vi "Rough TDMS Viewer.vi"() -> ()   [LabVIEW 2019, in "Report Viewer.lvlib" / "Report Viewer.lvclass"]
doc: "Defer all the request for panel update the panel list. This will improve the loading time."
uses:
  Report Viewer.lvclass
  Custom Controls/Browse Tools.ctl
  <vilib>/Utility/tdmsutil.llb/fileViewerConfigData.ctl
panel:
  out "TDMS File":string="Please using \"OPEN TDMS\" button to select tdms file."
  in  "Display Format":T1(ring)
  in  "Settings":bool
  in  "Properties / Values / Graph":T2(tab)=enum."Analog values (graph)"
  in  "Properties":i32(listbox)
  in  "Raw data values":i32(listbox)=-1
  out "Delta X (Time mS)":dbl
  out "Waveform Graph":waveform(dbl)[](graph)=[{"t0"=timestamp(0 s since 1904-01-01), "dt"=1.0, "Y"=[]}]
  out "Delta Y (Amplitude)":dbl
  in  "File contents":string[](tree)=["\"\u0000\u0000\u0000\u0002\u0000\u0000\u0000+Halt Mode Running_11:25:18.755 AM 11/6/2019\u0000\u0000\u0000\nPJB1_S CH0\""]
  in  "Open TDMS":bool
  in  "Save Graph":bool
  in  "Save Data":bool
  in  "Finished":bool
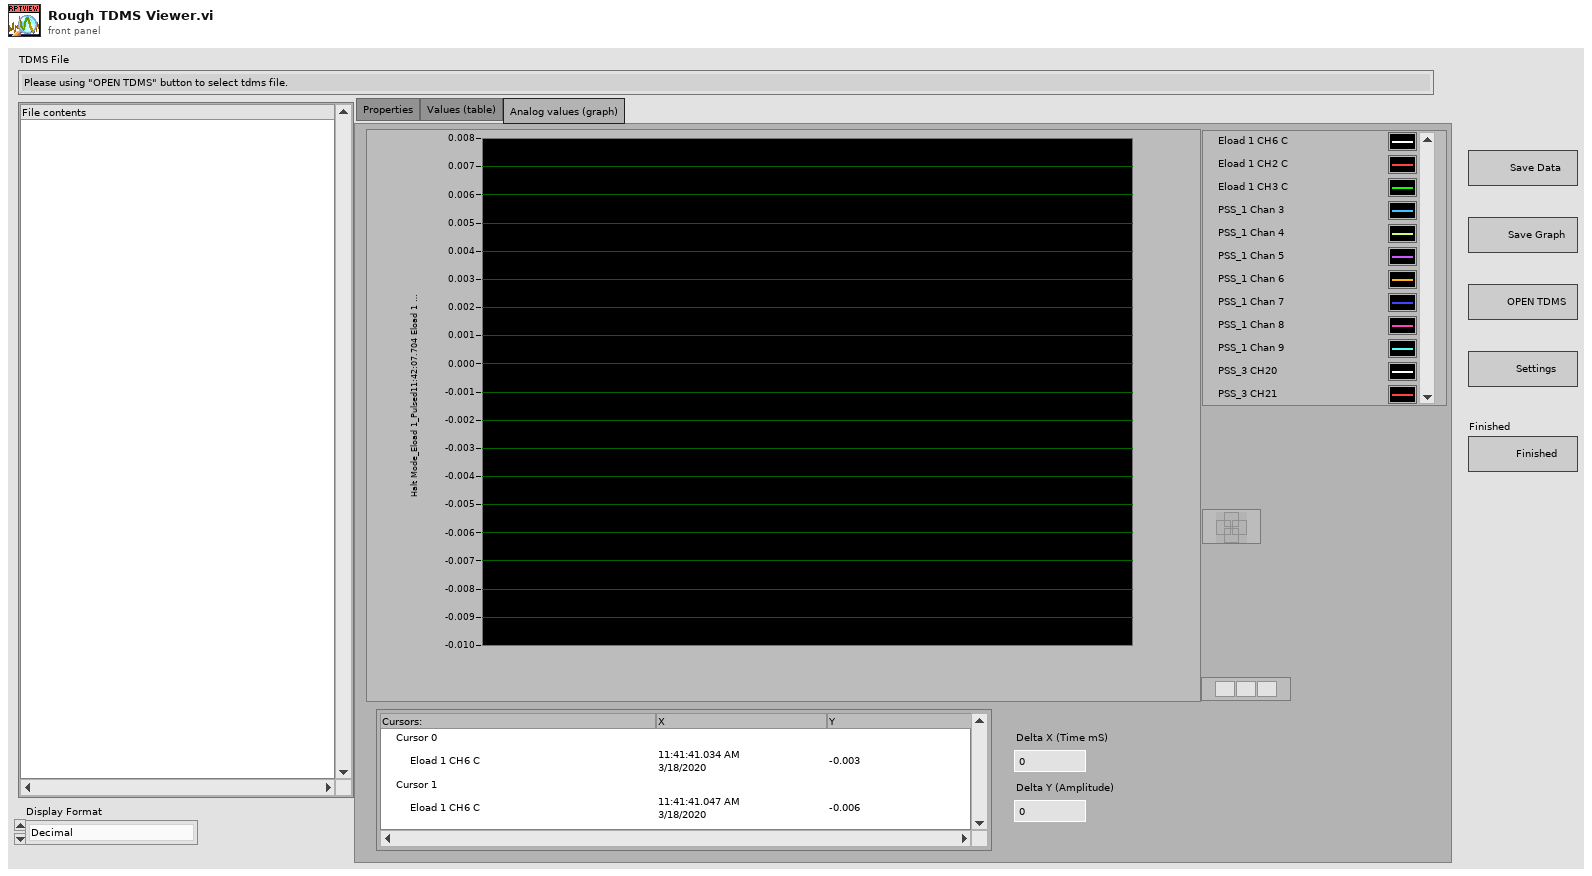
[diagram p1: front panel]
types:
  T1 = enum16{"Decimal", "Scientific", "Engineering", "Binary", "Octal", "Hexadecimal"}
  T2 = enum32{"Properties", "Values (table)", "Analog values (graph)"}
  T3 = enum32{"Invalid", "Standard", "Closed", "Hidden", "Minimized", "Maximized"}
  T4 = typedef "fileViewerConfigData.ctl" = cluster{"Show all (table)":bool, "Show all (graph)":bool, "limit (table)":u64, "limit (graph)":u64, "no show":bool, "start (table)":u64, "start (graph)":u64}
  T5 = typedef "Report Viewer.lvlib/Report Viewer.lvclass/Browse Tools.ctl" = cluster{"Group":string, "Channel":string, "TDMS View Cfg":T4}
  T6 = typedef "imagedata.ctl" = cluster{"image type":i32, "image depth":i32, "image":u8[], "mask":u8[], "colors":u32[], "Rectangle":cluster{"left":i16, "top":i16, "right":i16, "bottom":i16}}
  T7 = typedef "LVCursorListTypeDef.ctl" = cluster{"Name":string, "Color":u32, "Style":u8, "Point Style":u8, "Name Visible":bool, "Allow Drag":bool, "Cursor Mode":u32, "Plot":i32, "Index":i32, "Position":cluster{"X":dbl, "Y":dbl}, "X Scale":u32, "Y Scale":u32, "Watch Plots":i32[], "Watch All Plots":bool, "Plot Area":i32, "Label Offset":cluster{"X":dbl, "Y":dbl}}[]
  T8 = cluster{"Name":string, "Color":u32, "Style":u8, "Point Style":u8, "Name Visible":bool, "Allow Drag":bool, "Cursor Mode":u32, "Plot":i32, "Index":i32, "Position":cluster{"X":dbl, "Y":dbl}, "X Scale":u32, "Y Scale":u32, "Watch Plots":i32[], "Watch All Plots":bool, "Plot Area":i32, "Label Offset":cluster{"X":dbl, "Y":dbl}}
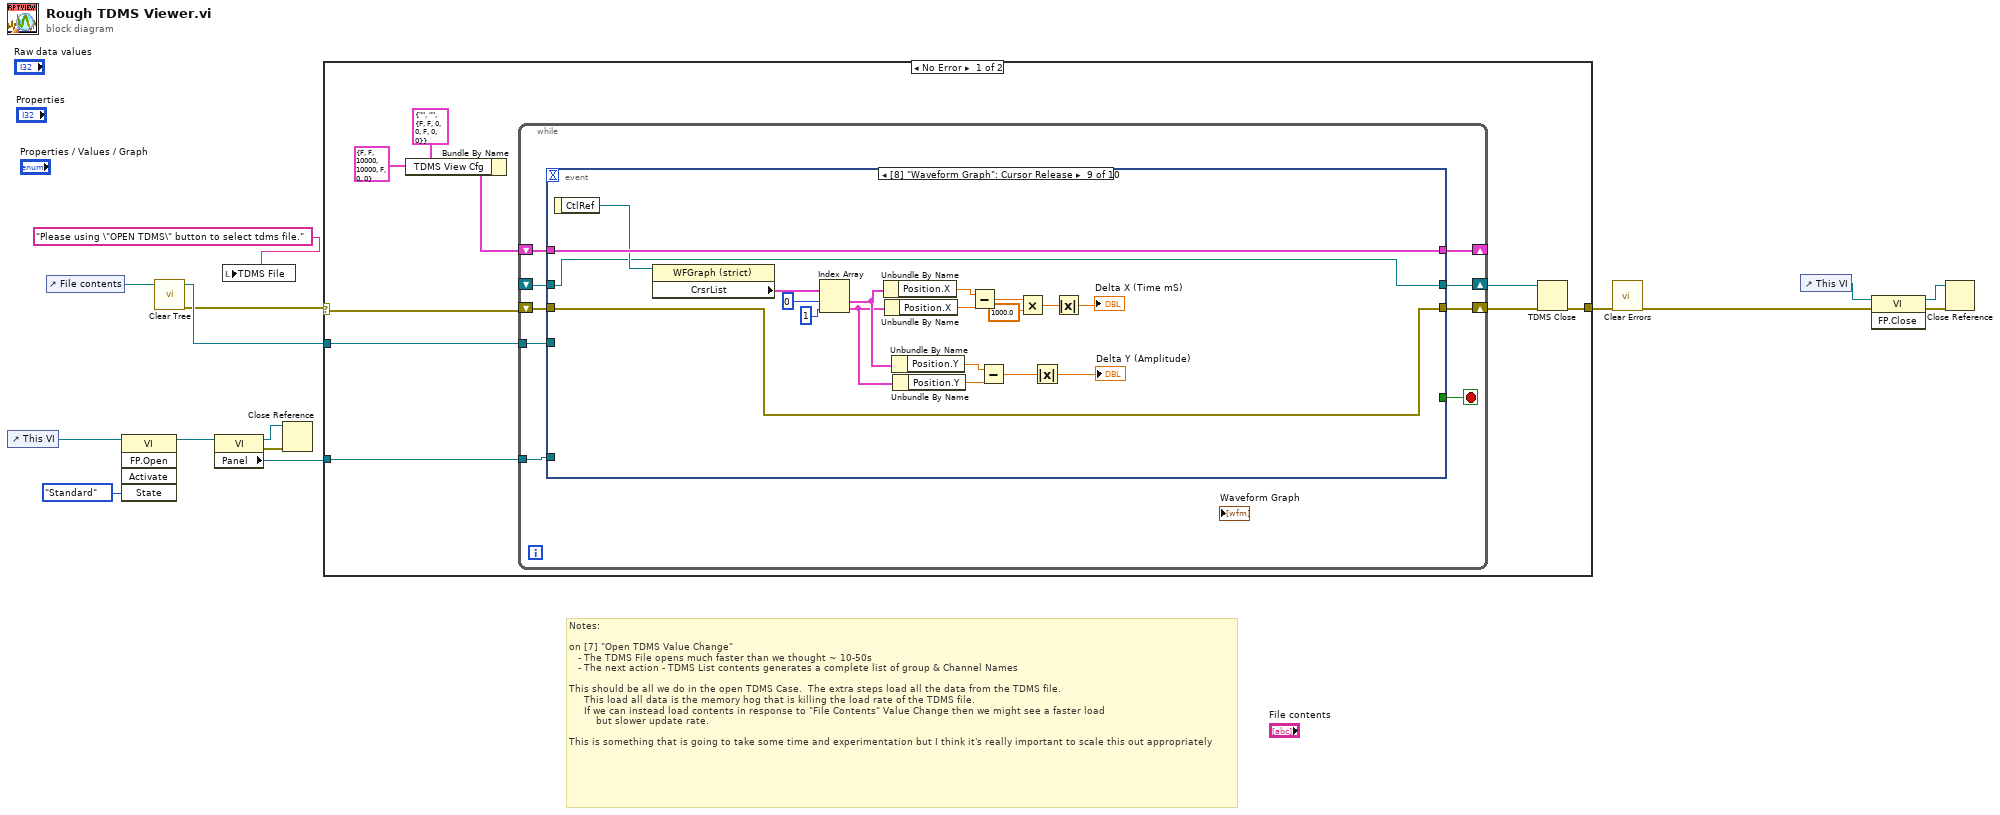
[diagram p0: block diagram]
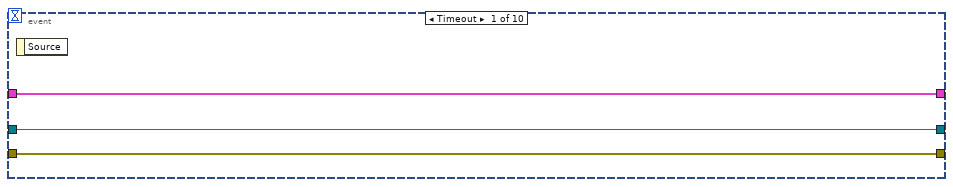
[diagram p2: hidden frame]
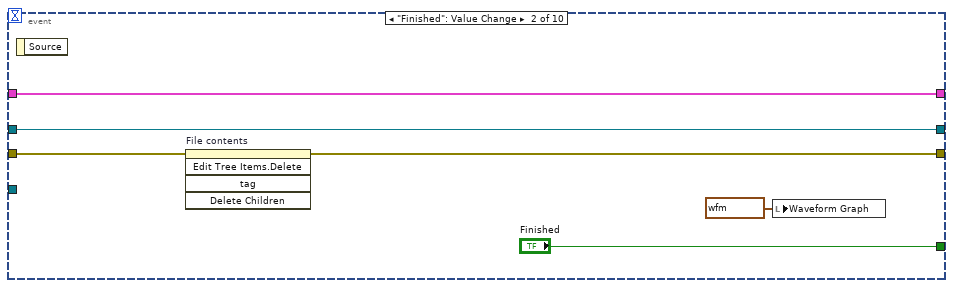
[diagram p3: hidden frame]
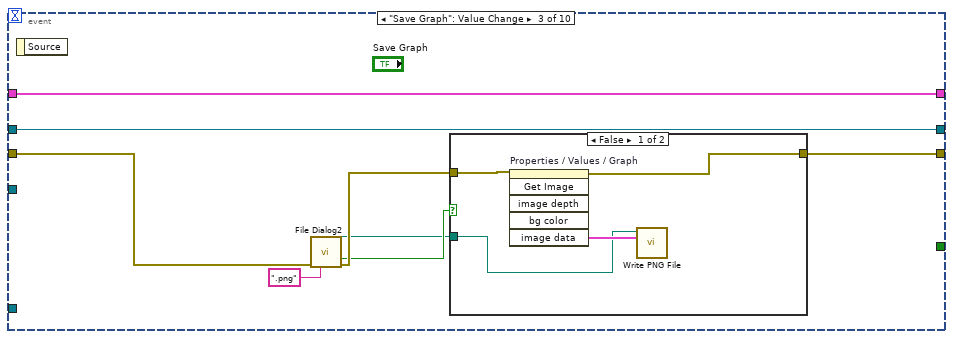
[diagram p4: hidden frame]
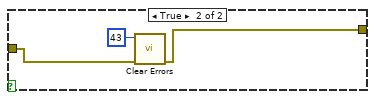
[diagram p5: hidden frame]
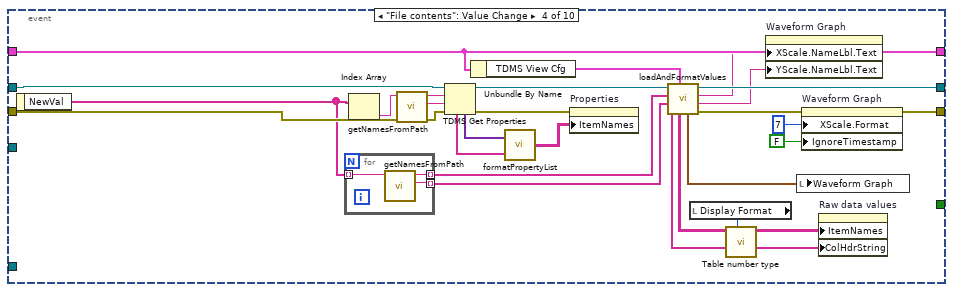
[diagram p6: hidden frame]
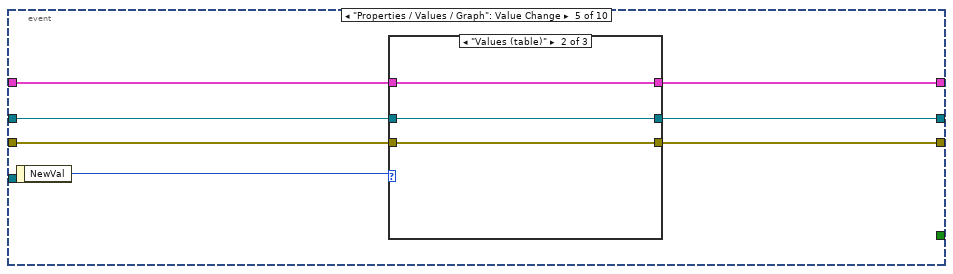
[diagram p7: hidden frame]
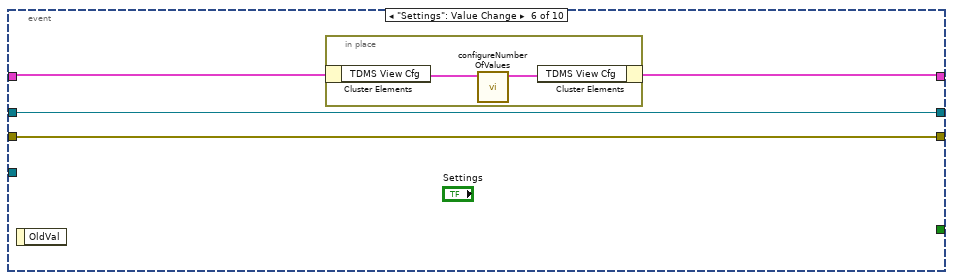
[diagram p10: hidden frame]
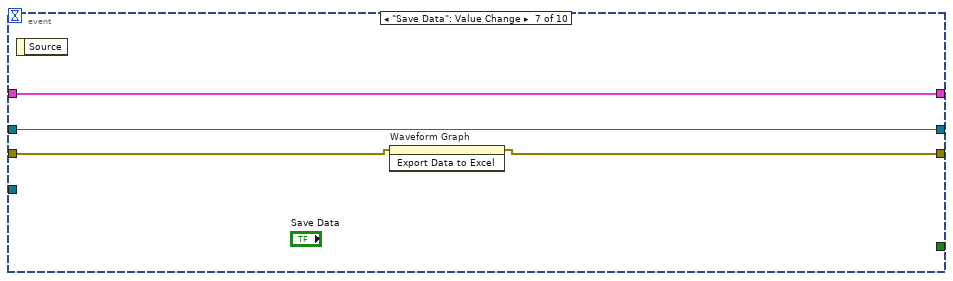
[diagram p11: hidden frame]
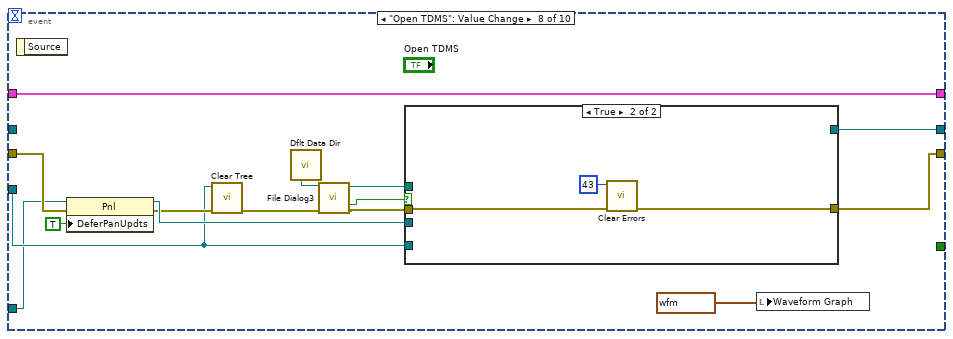
[diagram p12: hidden frame]
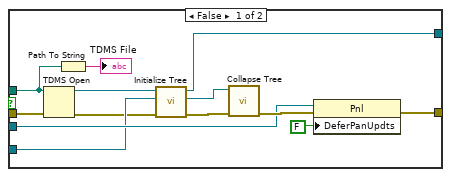
[diagram p13: hidden frame]
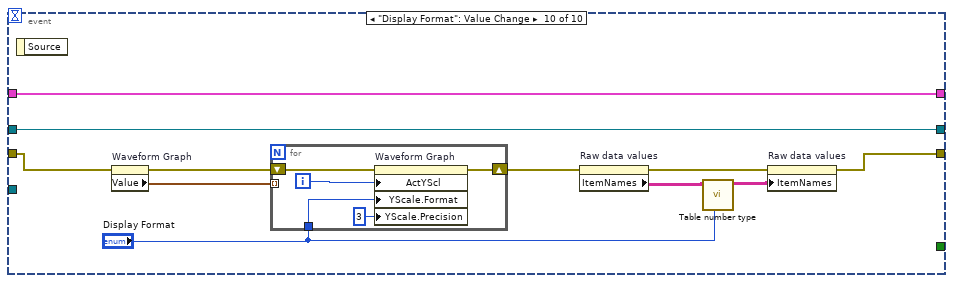
[diagram p14: hidden frame]
diagram:
  # "Notes:\n\non [7] \"Open TDMS Value Change\"\n   - The TDMS File opens much faster than we thought ~ 10-50s\n   - The next action - TDMS List contents generates a complete list of group & Channel Names\n\nThis should be all we do in the open TDMS Case.  The extra steps load all the data from the TDMS file.\n     This load all data is the memory hog that is killing the load rate of the TDMS file.  \n     If we can instead load contents in response to \"File Contents\" Value Change then we might see a faster load\n         but slower update rate.  \n\nThis is something that is going to take some time and experimentation but I think it's really important to scale this out appropriately"
  n1 = control-ref of="This VI"() -> (w13:refnum<vi>)
  n2 = control-ref of="File contents"() -> (w10:refnum<vi>)
  n3 = invoke class="VI" method="FP.Open"(reference=w13, "State"=T3."Standard") -> (reference out=w5:refnum<vi>)  [unwired: 3 in, 4 out]
  n4 = call "Clear Tree.vi"("reference"=w10) -> ("error out"=w8:errorcluster, "reference out"=w9:refnum<vi>)  [unwired: 9 in]
  n5 = property class="VI"(reference=w5) -> (reference out=w11:refnum<vi>, error out=w12:errorcluster, "Panel"=w6:refnum<vi>)  [unwired: 1 in]
  n6 = local write "TDMS File"("Please using \"OPEN TDMS\" button to select tdms file.") -> ()
  n7 = Close Reference(reference=w11, error in (no error)=w12) -> ()  [unwired: 1 out]
  n8 = case shown="No Error" w8 {
    selector: w8 -> [w17 w180]
    tunnel: [w24 w180] -> w15
    tunnel: w9 -> [w19 _]
    tunnel: w6 -> [w16 _]
    frame No Error {
      n9 = Bundle By Name(cluster=T5 {"Group"="", "Channel"="", "TDMS View Cfg"={"Show all (table)"=FALSE, "Show all (graph)"=FALSE, "limit (table)"=0, "limit (graph)"=0, "no show"=FALSE, "start (table)"=0, "start (graph)"=0}} ("Cluster"), "TDMS View Cfg"=T4 {"Show all (table)"=FALSE, "Show all (graph)"=FALSE, "limit (table)"=10000, "limit (graph)"=10000, "no show"=FALSE, "start (table)"=0, "start (graph)"=0} ("TDMS File Viewer Configuration")) -> (w21:T5)
      n10 = while {
        shift-right: [w31] -> w23
        shift-left: w17 -> [w32]
        shift-right: [w26] -> w18
        shift-left: _ -> [w33]
        shift-right: [w28] -> _
        shift-left: w21 -> [w29]
        tunnel: w19 -> [w27]
        tunnel: w16 -> [w25]
        stop <- w30 stop-if-true
        n11 = event shown="[8] \"Waveform Graph\": Cursor Release" {
          selector: _ -> [_ _ _ _ _ _ _ _ _ _]
          dyn-events: _ -> [_ _ _ _ _ _ _ _ _ _]
          timeout: _ -> [_ _ _ _ _ _ _ _ _ _]
          tunnel: w33 -> [w34 w39 w47 w63 w93 w104 w110 _ w150 w173]
          tunnel: w32 -> [w36 w37 w48 w84 w89 w105 w112 w121 w149 w166]
          tunnel: [w36 w37 w45 w67 w88 w105 w111 w126 w149 w171] -> w31
          tunnel: [_ "Finished" _ _ _ _ _ _ _ _] -> w30
          tunnel: w29 -> [w35 w40 w49 w75 w92 w107 w113 w128 w163 w174]
          tunnel: [w35 w40 w49 w75 w91 w106 w113 w128 w163 w174] -> w28
          tunnel: w27 -> [_ _ _ _ _ _ _ w117 _ _]
          tunnel: [w34 w39 w47 w64 w90 w104 w110 w125 w150 w173] -> w26
          tunnel: w25 -> [_ _ _ _ _ _ _ w116 _ _]
          event Timeout {
            n12 = event-data() -> ()  [unwired: 1 in, 1 out]
          }
          event "Finished": Value Change {
            n13 = event-data() -> ()  [unwired: 1 in, 1 out]
            n14 = invoke on="File contents" class="Tree (strict)" method="Edit Tree Items.Delete"(error in=w37) -> ()  [unwired: 4 in, 5 out]
            n15 = local write "Waveform Graph"(waveform(dbl)[] [{"t0"=timestamp(0 s since 1904-01-01), "dt"=1.0, "Y"=[]}] ("Waveform Graph")) -> ()
          }
          event "Save Graph": Value Change {
            n16 = event-data() -> ()  [unwired: 1 in, 1 out]
            n17 = call "File Dialog2"("error in"=w48, "pattern (all files)"=".png") -> ("selected path"=w43:path, "cancelled"=w44:bool, "error out"=w46:errorcluster)  [unwired: 10 in, 1 out]
            n18 = case shown="False" w44 {
              tunnel: [w53 w54] -> w45
              tunnel: w46 -> [w52 w55]
              tunnel: w43 -> [w50 _]
              frame False {
                n19 = invoke on="Properties / Values / Graph" class="TabCtl (strict)" method="Get Image"(error in=w52) -> (error out=w53:errorcluster, "image data"=w51:T6)  [unwired: 5 in, 4 out]
                n20 = call <vilib>:"Write PNG File.vi"("image data"=w51, "path to PNG file"=w50) -> ()  [unwired: 8 in, 2 out]
              }
              frame True {
                n21 = call <vilib>:"Clear Errors.vi"("error in (no error)"=w55, "specific error code to clear (0: all)"=43) -> ("error out"=w54:errorcluster)  [unwired: 4 in, 1 out]
              }
            }
          }
          event "File contents": Value Change {
            n22 = event-data() -> ("NewVal"=w72:string[])  [unwired: 1 in]
            n23 = for {
              tunnel: w72 -> [w87] mode=indexing
              tunnel: [w86] -> w71 mode=indexing
              tunnel: [w85] -> w70 mode=indexing
              n24 = call <vilib>:"getNamesFromPath.vi"("tree path"=w87) -> ("channel"=w85:string, "group"=w86:string)  [unwired: 1 in, 4 out]
            }
            n25 = Index Array(array=w72) -> (element=w76:string)  [unwired: 1 in]
            n26 = call <vilib>:"getNamesFromPath.vi"("error in (no error)"=w84, "tree path"=w76) -> ("error out"=w83:errorcluster, "channel"=w81:string, "group"=w82:string)  [unwired: 3 out]
            n27 = TDMS Get Properties(8:w83, 9:w81, 10:w82, 11:w63) -> (0:w77:errorcluster, 3:w73:refnum<k34>, 4:w80:variant[], 6:w79:string[])  [unwired: 4 out]
            n28 = Unbundle By Name(w75) -> ("TDMS View Cfg"=w74:T4)
            n29 = call <vilib>:"formatPropertyList.vi"("property names"=w79, "property values"=w80) -> ("strings"=w78:string[][])
            n30 = property on="Properties" class="MCListbox (strict)"(error in=w77, "ItemNames"=w78) -> ()  [unwired: 1 in, 2 out]
            n31 = call <vilib>:"loadAndFormatValues.vi"("configuration"=w74, "channel names"=w70, "group names"=w71, "tdms file"=w73) -> ("error out"=w68:errorcluster, "graph y names"=w61:string, "graph x names"=w62:string, "tdms file out"=w64:refnum<k34>, "waveform values"=w57:waveform(dbl)[], "table values"=w59:string[][], "table headers"=w69:string[])  [unwired: 1 in]
            n32 = local read "Display Format"() -> (w58:T1)
            n33 = call "Table number type.vi"("Y Scale.Display Format:Format"=w58, "Item Names in"=w59) -> ("Item Names out"=w60:string[][])  [unwired: 9 in]
            n34 = property on="Waveform Graph" class="WFGraph (strict)"("XScale.NameLbl.Text"=w62, "YScale.NameLbl.Text"=w61) -> ()  [unwired: 2 in, 2 out]
            n35 = local write "Waveform Graph"(w57) -> ()
            n36 = property on="Waveform Graph" class="WFGraph (strict)"(error in=w68, "XScale.Format"=u8 7 ("X Scale.Display Format:Format"), "IgnoreTimestamp"=FALSE ("Ignore Timestamp")) -> (error out=w67:errorcluster)  [unwired: 1 in, 1 out]
            n37 = property on="Raw data values" class="MCListbox (strict)"("ItemNames"=w60, "ColHdrString"=w69) -> ()  [unwired: 2 in, 2 out]
          }
          event "Properties / Values / Graph": Value Change {
            n38 = event-data() -> ("NewVal"=w94:T2)  [unwired: 1 in]
            n39 = case shown="\"Values (table)\"" w94 {
              tunnel: w93 -> [w97 w99 w102]
              tunnel: [w97 w99 w102] -> w90
              tunnel: w92 -> [w96 w100 w103]
              tunnel: [w96 w100 w103] -> w91
              tunnel: w89 -> [w95 w98 w101]
              tunnel: [w95 w98 w101] -> w88
              frame "Properties", Default {
              }
              frame "Values (table)" {
              }
              frame "Analog values (graph)" {
              }
            }
          }
          event "Settings": Value Change {
            n40 = event-data() -> ()  [unwired: 1 in, 1 out]
            n41 = in-place {
              n42 = in-place-cluster #1(w107) -> ("TDMS View Cfg"=w109:T4)
              n43 = call <vilib>:"configureNumberOfValues.vi"("TDMS File Viewer Configuration"=w109) -> ("TDMS File Viewer Configuration Out"=w108:T4)  [unwired: 10 out]
              n44 = in-place-cluster #1("TDMS View Cfg"=w108) -> (w106:T5)
            }
          }
          event "Save Data": Value Change {
            n45 = event-data() -> ()  [unwired: 1 in, 1 out]
            n46 = invoke on="Waveform Graph" class="WFGraph (strict)" method="Export Data to Excel"(error in=w112) -> (error out=w111:errorcluster)  [unwired: 2 in, 2 out]
          }
          event "Open TDMS": Value Change {
            n47 = event-data() -> ()  [unwired: 1 in, 1 out]
            n48 = property class="Pnl"(reference=w116, error in=w121, "DeferPanUpdts"=TRUE ("Defer Panel Updates")) -> (reference out=w120:refnum<vi>, error out=w119:errorcluster)
            n49 = call "Clear Tree.vi"("error in"=w119, "reference"=w117) -> ("error out"=w118:errorcluster)  [unwired: 8 in, 1 out]
            n50 = call <vilib>:"Dflt Data Dir.vi"() -> ("App:Default Data Directory"=w127:path)
            n51 = call "File Dialog3"("start path"=w127, "error in"=w118) -> ("selected path"=w123:path, "cancelled"=w114:bool, "error out"=w115:errorcluster)  [unwired: 10 in, 1 out]
            n52 = case shown="True" w114 {
              tunnel: [w137 w143] -> w126
              tunnel: [w136 _] -> w125
              tunnel: w123 -> [w134 _]
              tunnel: w120 -> [w133 _]
              tunnel: w117 -> [w132 _]
              tunnel: w115 -> [w131 w144]
              frame False {
                n53 = TDMS Open(8:w131, 11:w134) -> (0:w130:errorcluster, 3:w129:refnum<k34>)  [unwired: 5 in]
                n54 = Path To String(path=w134) -> (string=→"TDMS File":string)
                n55 = call "Initialize Tree.vi"("error in"=w130, "reference"=w132, "tdms file"=w129) -> ("error out"=w139:errorcluster, "tree reference out"=w140:refnum<vi>, "tdms file out"=w136:refnum<k34>)  [unwired: 6 in]
                n56 = call "Collapse Tree.vi"("error in (no error)"=w139, "Tree Ref in"=w140) -> ("error out"=w138:errorcluster)  [unwired: 8 in, 1 out]
                n57 = property class="Pnl"(reference=w133, error in=w138, "DeferPanUpdts"=FALSE ("Defer Panel Updates")) -> (error out=w137:errorcluster)  [unwired: 1 out]
              }
              frame True {
                n58 = call <vilib>:"Clear Errors.vi"("error in (no error)"=w144, "specific error code to clear (0: all)"=43) -> ("error out"=w143:errorcluster)  [unwired: 4 in, 1 out]
              }
            }
            n59 = local write "Waveform Graph"(waveform(dbl)[] [{"t0"=timestamp(0 s since 1904-01-01), "dt"=1.0, "Y"=[]}] ("Waveform Graph")) -> ()
          }
          event "Waveform Graph": Cursor Release {
            n60 = event-data() -> ("CtlRef"=w155:refnum<vi>)  [unwired: 1 in]
            n61 = property on="Property Node" class="WFGraph (strict)"(reference=w155) -> ("CrsrList"=w162:T7)  [unwired: 1 in, 2 out]
            n62 = Index Array(array=w162, index #1=0 ("index"), index #2=1 ("index")) -> (element #1=w152:T8, element #2=w151:T8)
            n63 = Unbundle By Name(w152) -> ("Position.X"=w158:dbl)
            n64 = Unbundle By Name(w151) -> ("Position.X"=w159:dbl)
            n65 = Unbundle By Name(w152) -> ("Position.Y"=w153:dbl)
            n66 = Unbundle By Name(w151) -> ("Position.Y"=w154:dbl)
            n67 = Subtract(x=w158, y=w159) -> (x-y=w157:dbl)
            n68 = Subtract(x=w153, y=w154) -> (x-y=w146:dbl)
            n69 = Multiply(x=w157, y=1000.0) -> (x*y=w148:dbl)
            n70 = Absolute Value(x=w146) -> (abs(x)=→"Delta Y (Amplitude)":dbl)
            n71 = Absolute Value(x=w148) -> (abs(x)=→"Delta X (Time mS)":dbl)
          }
          event "Display Format": Value Change {
            n72 = event-data() -> ()  [unwired: 1 in, 1 out]
            n73 = property on="Waveform Graph" class="WFGraph (strict)"(error in=w166) -> (error out=w165:errorcluster, "Value"=w164:waveform(dbl)[])  [unwired: 1 in, 1 out]
            n74 = for {
              tunnel: "Display Format" -> [w178]
              shift-right: [w179] -> w172
              shift-left: w165 -> [w177]
              tunnel: w164 -> [_] mode=indexing
              i -> [w176]
              n75 = property on="Waveform Graph" class="WFGraph (strict)"(error in=w177, "ActYScl"=w176, "YScale.Format"=w178, "YScale.Precision"=u8 3 ("Y Scale.Display Format:Precision")) -> (error out=w179:errorcluster)  [unwired: 1 in, 1 out]
            }
            n76 = property on="Raw data values" class="MCListbox (strict)"(error in=w172) -> (error out=w170:errorcluster, "ItemNames"=w169:string[][])  [unwired: 1 in, 1 out]
            n77 = call "Table number type.vi"("Y Scale.Display Format:Format"="Display Format", "Item Names in"=w169) -> ("Item Names out"=w168:string[][])  [unwired: 9 in]
            n78 = property on="Raw data values" class="MCListbox (strict)"(error in=w170, "ItemNames"=w168) -> (error out=w171:errorcluster)  [unwired: 1 in, 1 out]
          }
        }
      }
      n79 = TDMS Close(8:w23, 11:w18) -> (0:w24:errorcluster)  [unwired: 1 out]
    }
    frame Error {
    }
  }
  n80 = call <vilib>:"Clear Errors.vi"("error in (no error)"=w15) -> ("error out"=w14:errorcluster)  [unwired: 5 in, 1 out]
  n81 = control-ref of="This VI"() -> (w3:refnum<vi>)
  n82 = invoke class="VI" method="FP.Close"(reference=w3, error in=w14) -> (reference out=w2:refnum<vi>, error out=w1:errorcluster)  [unwired: 1 in, 1 out]
  n83 = Close Reference(reference=w2, error in (no error)=w1) -> ()  [unwired: 1 out]
